vi "ATR FPGA arbiter.vi"(8 "User input valid":bool, 9 "User ATR state":u8, 10 "RegBus input valid":bool, 11 "RegBus ATR state":u8) -> (3 "ATR out":u8)   [LabVIEW 2023]
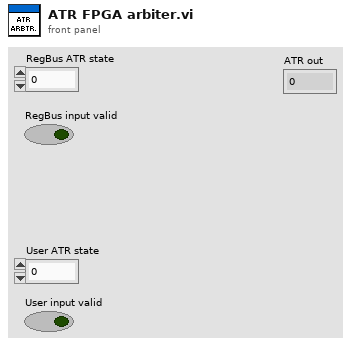
[diagram p1: front panel]
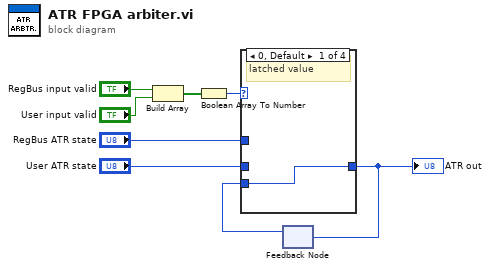
[diagram p0: block diagram]
diagram:
  n1 = Build Array("RegBus input valid", "User input valid") -> (w3:bool[])
  n2 = Boolean Array To Number(Boolean array=w3) -> (number=w4:u32)
  n3 = feedback #1() -> (w7:u8)  [unwired: 1 in]
  n4 = case shown="0, Default" w4 {
    tunnel: "RegBus ATR state" -> [_ w10 _ _]
    tunnel: "User ATR state" -> [_ _ w11 w12]
    tunnel: w7 -> [w9 _ _ _]
    tunnel: [w9 w10 w11 w12] -> w8
    frame 0, Default {
      # "latched value"
    }
    frame 1 {
      # "RegBus"
    }
    frame 2 {
      # "User"
    }
    frame 3 {
      # "User wins"
    }
  }
  "ATR out" <- w8
  n5 = feedback-in #1(w8) -> ()
